vi "Drehzahl Setzen.vi"(8 "Error In":errorcluster caption="Fehler (Eingang)", 10 "Drehzahl U/Min":dbl, 11 "connection_ID_In":refnum<k5>) -> (0 "Error Out":errorcluster caption="Fehler (Ausgang)", 3 "connection_ID_Out":refnum<k5>)   [LabVIEW 2019, in "Motor Treiber.lvlib"]
doc: "Dieses VI sendet einen neuen Sollwert zu dem Thermotat. Der Therostat erlaubt nur Werte zweischen 0 und 100%. Wenn der Wert außerhalb des Bereiches liegt, liefert die Funktion einen fehler als Rückgabe."
uses:
  Motor Treiber.lvlib
  SubVIs/Simulationsvariable.vi
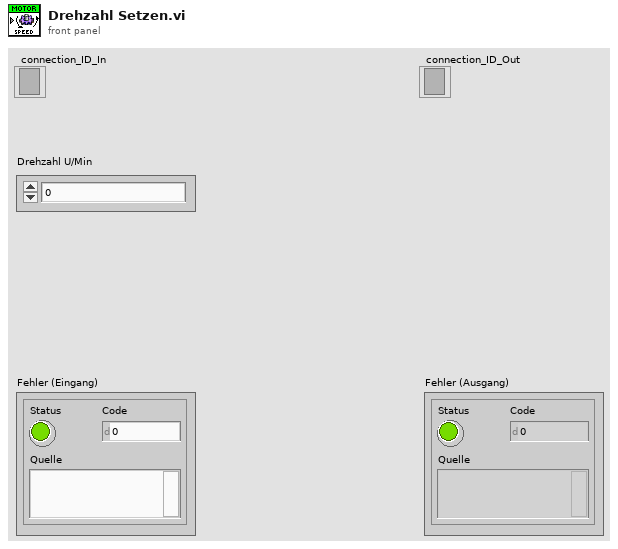
[diagram p1: front panel]
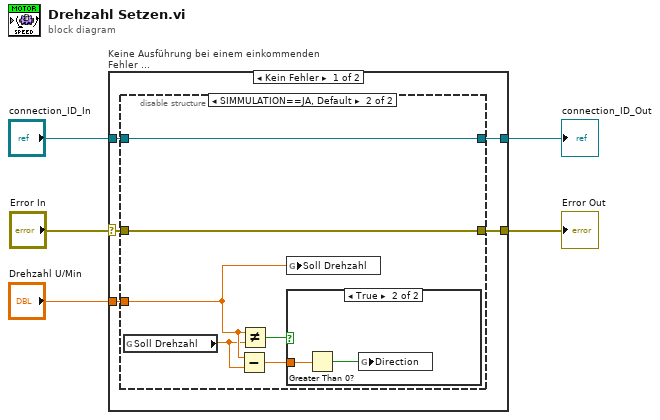
[diagram p0: block diagram]
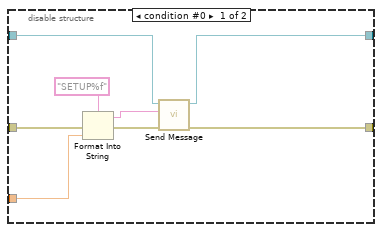
[diagram p2: hidden frame]
diagram:
  n1 = case "Keine Ausführung bei einem einkommenden Fehler ..." shown="Kein Fehler" "Error In" {
    selector: "Error In" -> [w10 w28]
    tunnel: [w7 w28] -> w4
    tunnel: "connection_ID_In" -> [w9 w27]
    tunnel: [w8 w27] -> w2
    tunnel: "Drehzahl U/Min" -> [w6 _]
    frame No Error {
      n2 = disable-structure shown="SIMMULATION==JA, Default" {
        disable-tunnel: w10 -> [w18 w24]
        disable-tunnel: w9 -> [w17 w23]
        disable-tunnel: [w16 w23] -> w8
        disable-tunnel: [w15 w24] -> w7
        disable-tunnel: w6 -> [w11 w21]
        frame condition #0 {
          n3 = Format Into String(format string="SETUP%f" ("Nachricht"), error in=w18, w11) -> (resulting string=w13:string, error out=w14:errorcluster)  [unwired: 1 in]
          n4 = call "Send Message.vi"("Error In"=w14, "Nachricht"=w13, "connection_ID_In"=w17) -> ("Error Out"=w15:errorcluster, "connection_ID_Out"=w16:refnum<k5>)  [unwired: 7 in]
        }
        frame condition #1 (active) {
          n5 = global read "Simulationsvariable.vi" "Soll Drehzahl"() -> (w20:dbl)
          n6 = Subtract(x=w21, y=w20) -> (x-y=w19:dbl)
          n7 = Not Equal?(x=w21, y=w20) -> (x != y?=w22:bool)
          n8 = global write "Simulationsvariable.vi" "Soll Drehzahl"(w21) -> ()
          n9 = case shown="True" w22 {
            tunnel: w19 -> [_ w26]
            frame False {
            }
            frame True {
              n10 = Greater Than 0?(x=w26) -> (x > 0?=w25:bool)
              n11 = global write "Simulationsvariable.vi" "Direction"(w25) -> ()
            }
          }
        }
      }
    }
    frame Error {
    }
  }
  "Error Out" <- w4
  "connection_ID_Out" <- w2
